vi "日志、报警信息存储 (子VI).vi"() -> ()   [LabVIEW 2016, in "超标留样集成.lvlib" / "ESTD1200.lvlib"]
uses:
  ESTD1200.lvlib
  <vilib>/ptbypt/NI_PtbyPt.lvlib
panel:
  out "采样器状态":u16(ring) items=["空闲", "忙碌"]
  out "状态告警区":T1 {"告警代码" items=["无告警", "通讯异常(采样器与工控机通讯)", "滑台电机异常(过温/过流)", "蠕动泵异常(过温/过流)", "转盘电机异常(过温/过流)", "编码器异常", "转盘原点传感器异常", "滑台原点传感器异常", "冰箱温度异常", "冰箱通讯异常", "门禁锁异常", "串口屏通讯异常", "SD卡异常告警", "Flash异常告警(W25Q32)", "留样失败", "满瓶告警", "复位异常"]; "采样模式" items=["定时采样", "外控采样", "时间等比", "流量等比", "液位等比"]; "当前进程" items=["待机", "电机复位", "采样瓶转到采样区", "采样瓶排空", "采样泵管润洗", "采样瓶再排空", "采样", "采样泵反转排空管路", "取样瓶转到取样区"]}
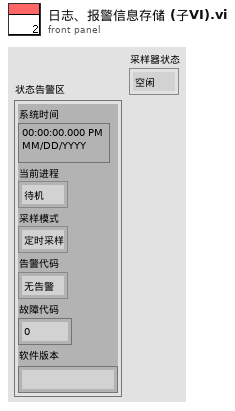
[diagram p1: front panel]
types:
  T1 = cluster{"系统时间":timestamp, "当前进程":u16, "采样模式":u16, "告警代码":u16, "故障代码":u16, "软件版本":string}
  T2 = cluster{"时间标识":timestamp, "设备":string, "日志信息":string, "流程参数":string}
  T3 = cluster{"时间标识":timestamp, "设备":string, "日志信息":string}
  T4 = cluster{"采样器状态":u16, "采样模式":u16, "瓶数":u16, "采样量":u16, "当前瓶号":u16, "当前进程":u16, "采样瓶状态":cluster{"1号瓶":bool, "2号瓶":bool, "3号瓶":bool, "4号瓶":bool, "5号瓶":bool, "6号瓶":bool, "7号瓶":bool, "8号瓶":bool, "9号瓶":bool, "10号瓶":bool, "11号瓶":bool, "12号瓶":bool}, "门锁状态":bool, "冰箱当前温度":sgl, "系统时间":timestamp}
  T5 = cluster{"当前瓶号":u16, "瓶数":u16, "采样量":u16, "采样模式":u16, "整点定时时间":cluster{"1":bool, "2":bool, "3":bool, "4":bool, "5":bool, "6":bool, "7":bool, "8":bool, "9":bool, "10":bool, "11":bool, "12":bool, "13":bool, "14":bool, "15":bool, "16":bool, "17":bool, "19":bool, "19":bool, "20":bool, "21":bool, "22":bool, "23":bool, "24":bool}, "氨氮":sgl, "总磷":sgl, "总氮":sgl, "CODMn":sgl, "CODCr":sgl, "PH":sgl, "溶解氧":sgl, "时间等比采样间隔":u16, "流量等比采样间隔":sgl, "4mA流量":sgl, "20mA流量":sgl, "当前流量":sgl, "液位等比采样间隔":sgl, "4mA液位":sgl, "20mA液位":sgl, "当前液位":sgl}
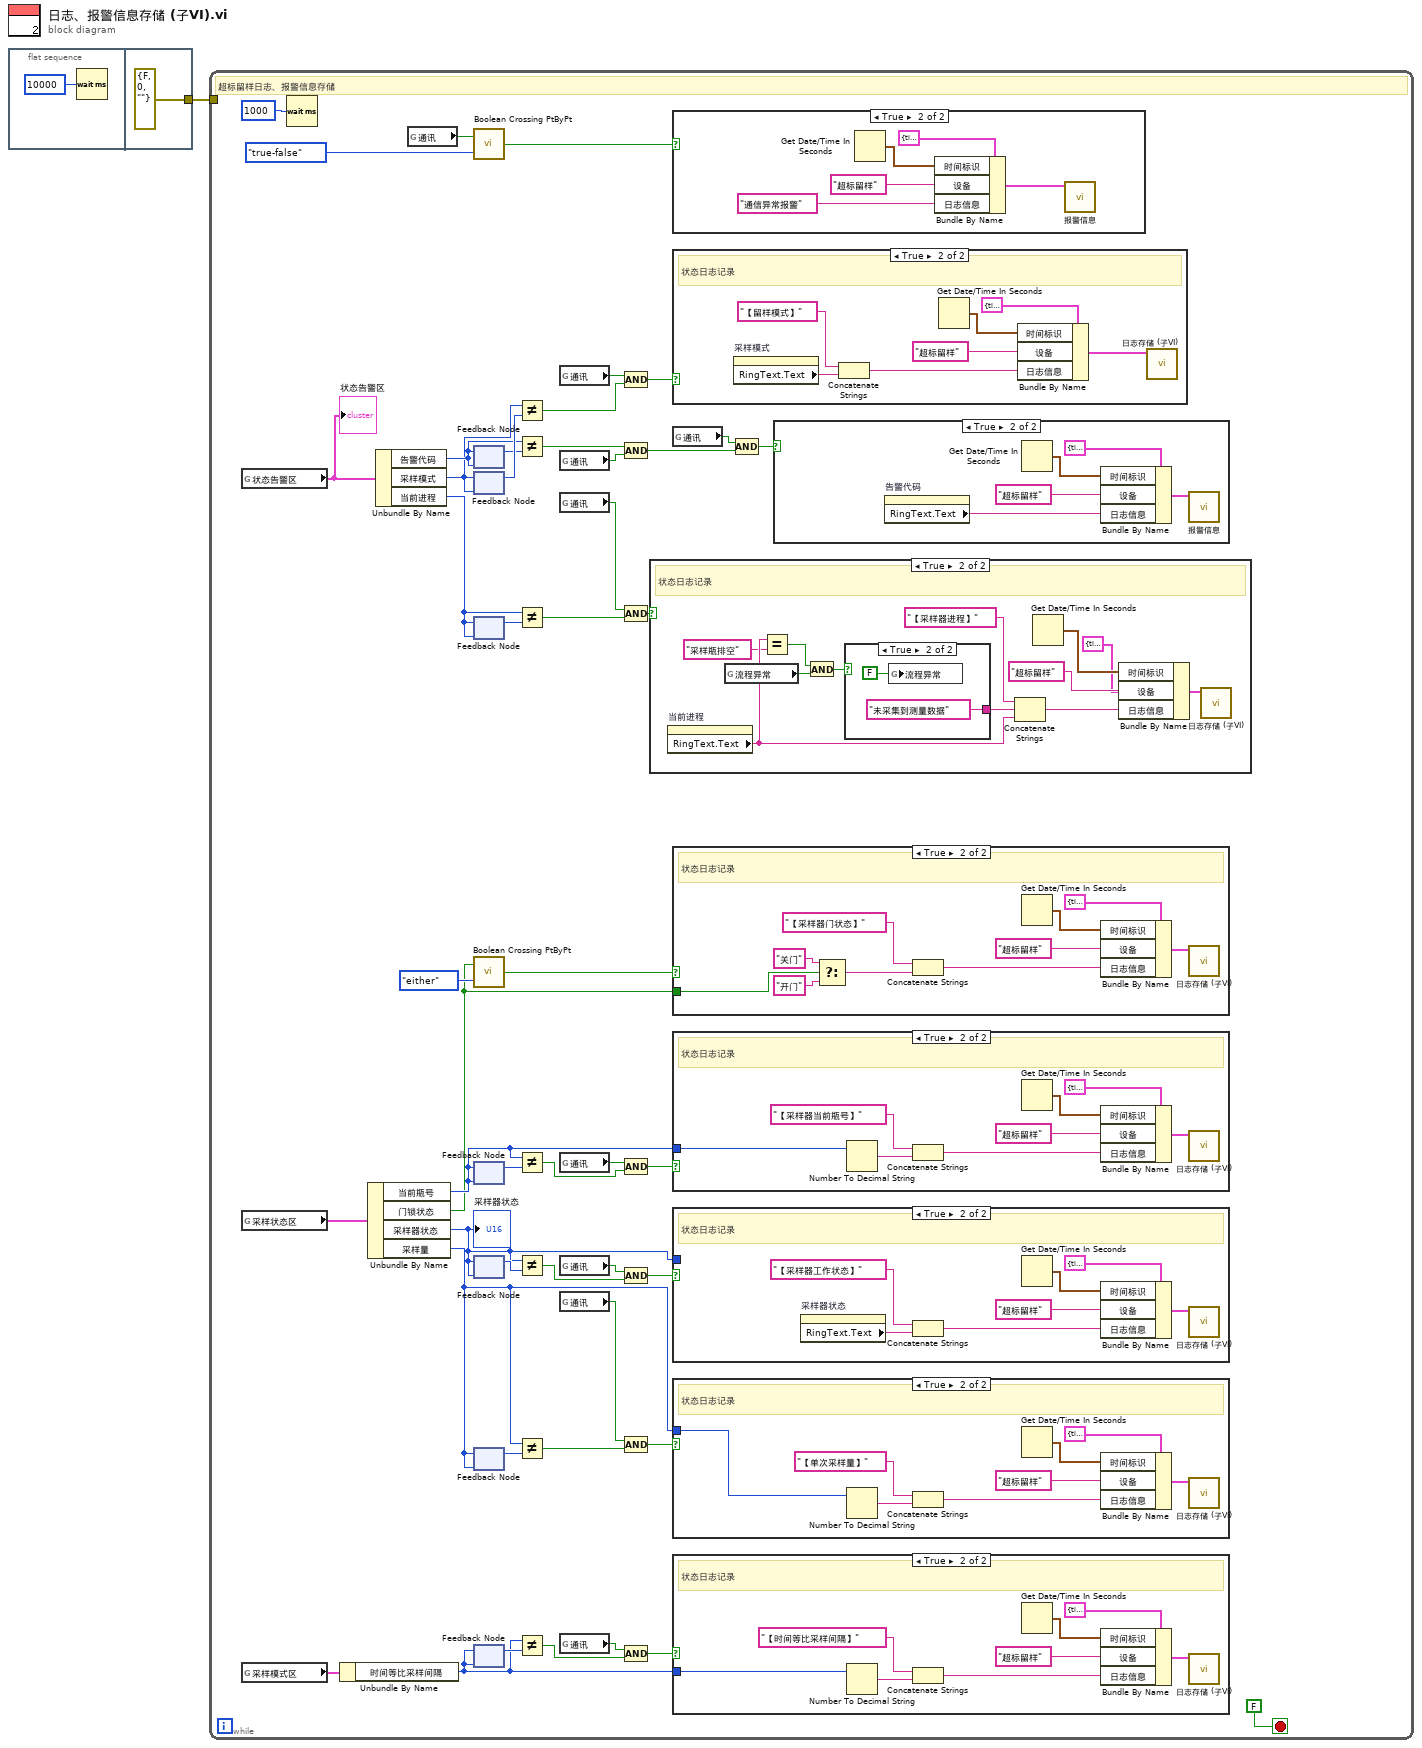
[diagram p0: block diagram]
diagram:
  n1 = flat-sequence {
    tunnel: [errorcluster {"status"=FALSE, "code"=0, "source"=""} ("错误常量")] -> w1
    frame #0 {
      n2 = Wait (ms)(milliseconds to wait=u32 10000 ("等待时间（毫秒）")) -> ()  [unwired: 1 out]
    }
    frame #1 {
    }
  }
  n3 = while {
    tunnel: w1 -> [_]
    stop <- FALSE stop-if-true
    # "超标留样日志、报警信息存储"
    n4 = global read "超标留样全局.vi" "状态告警区"() -> (w16:T1)
    "状态告警区" <- w16
    n5 = global read "超标留样全局.vi" "采样状态区"() -> (w13:T4)
    n6 = global read "超标留样全局.vi" "采样模式区"() -> (w6:T5)
    n7 = Wait (ms)(milliseconds to wait=u32 1000 ("等待时间（毫秒）")) -> ()  [unwired: 1 out]
    n8 = Unbundle By Name(w6) -> ("时间等比采样间隔"=w5:u16)
    n9 = Unbundle By Name(w13) -> ("当前瓶号"=w12:u16, "门锁状态"=w9:bool, "采样器状态"=w8:u16, "采样量"=w7:u16)
    "采样器状态" <- w8
    n10 = Unbundle By Name(w16) -> ("告警代码"=w17:u16, "采样模式"=w15:u16, "当前进程"=w14:u16)
    n11 = global read "超标留样全局.vi" "通讯"() -> (w20:bool)
    n12 = call <vilib>:"Boolean Crossing PtByPt.vi"("direction"=enum16{"either", "false-true", "true-false"}."true-false", "input"=w20) -> ("crossing"=w18:bool)  [unwired: 1 in]
    n13 = feedback #1(w17) -> (w4:u16)
    n14 = feedback-in #1(w17) -> ()
    n15 = feedback #2(w15) -> (w43:u16)
    n16 = feedback-in #2(w15) -> ()
    n17 = feedback #3(w14) -> (w49:u16)
    n18 = feedback-in #3(w14) -> ()
    n19 = call <vilib>:"Boolean Crossing PtByPt.vi"("direction"=enum16{"either", "false-true", "true-false"}."either", "input"=w9) -> ("crossing"=w10:bool)  [unwired: 1 in]
    n20 = feedback #4(w12) -> (w48:u16)
    n21 = feedback-in #4(w12) -> ()
    n22 = feedback #5(w8) -> (w47:u16)
    n23 = feedback-in #5(w8) -> ()
    n24 = feedback #6(w7) -> (w46:u16)
    n25 = feedback-in #6(w7) -> ()
    n26 = feedback #7(w5) -> (w42:u16)
    n27 = feedback-in #7(w5) -> ()
    n28 = Not Equal?(x=w15, y=w43) -> (x != y?=w34:bool)
    n29 = Not Equal?(x=w17, y=w4) -> (x != y?=w39:bool)
    n30 = Not Equal?(x=w14, y=w49) -> (x != y?=w35:bool)
    n31 = Not Equal?(x=w12, y=w48) -> (x != y?=w30:bool)
    n32 = Not Equal?(x=w8, y=w47) -> (x != y?=w28:bool)
    n33 = Not Equal?(x=w7, y=w46) -> (x != y?=w25:bool)
    n34 = Not Equal?(x=w5, y=w42) -> (x != y?=w21:bool)
    n35 = global read "超标留样全局.vi" "通讯"() -> (w38:bool)
    n36 = global read "超标留样全局.vi" "通讯"() -> (w41:bool)
    n37 = global read "超标留样全局.vi" "通讯"() -> (w37:bool)
    n38 = global read "超标留样全局.vi" "通讯"() -> (w32:bool)
    n39 = global read "超标留样全局.vi" "通讯"() -> (w29:bool)
    n40 = global read "超标留样全局.vi" "通讯"() -> (w26:bool)
    n41 = global read "超标留样全局.vi" "通讯"() -> (w23:bool)
    n42 = Compound Arithmetic op=AND ("复合运算")(w38, w34) -> (w33:bool)
    n43 = Compound Arithmetic op=AND ("复合运算")(w39, w41) -> (w40:bool)
    n44 = Compound Arithmetic op=AND ("复合运算")(w37, w35) -> (w36:bool)
    n45 = Compound Arithmetic op=AND ("复合运算")(w32, w30) -> (w31:bool)
    n46 = Compound Arithmetic op=AND ("复合运算")(w29, w28) -> (w27:bool)
    n47 = Compound Arithmetic op=AND ("复合运算")(w26, w25) -> (w24:bool)
    n48 = Compound Arithmetic op=AND ("复合运算")(w23, w21) -> (w22:bool)
    n49 = case shown="True" w36 {
      frame False {
      }
      frame True {
        # "状态日志记录"
        n50 = property on="当前进程" class="Ring (strict)"() -> ("RingText.Text"=w115:string)  [unwired: 2 in, 2 out]
        n51 = global read "串口参数断电保存全局变量.vi" "流程异常"() -> (w112:bool)
        n52 = Equal?(x=w115, y="采样瓶排空") -> (x = y?=w113:bool)
        n53 = And(x=w113, y=w112) -> (x .and. y?=w111:bool)
        n54 = case shown="True" w111 {
          tunnel: [_ "未采集到测量数据" ("t")] -> w110
          frame False {
          }
          frame True {
            n55 = global write "串口参数断电保存全局变量.vi" "流程异常"(FALSE) -> ()
          }
        }
        n56 = Concatenate Strings("【采样器进程】" ("日志信息"), w110, w115) -> (w121:string)
        n57 = Get Date/Time In Seconds() -> (seconds since 1Jan1904=w119:timestamp)
        n58 = Bundle By Name(cluster=T2 {"时间标识"=timestamp(0 s since 1904-01-01), "设备"="", "日志信息"="", "流程参数"=""} ("data in"), "时间标识"=w119, "设备"="超标留样", "日志信息"=w121) -> (w116:T2)
        n59 = call "日志存储 (子VI).vi"("data in"=w116) -> ()  [unwired: 11 in]
      }
    }
    n60 = case shown="True" w18 {
      frame False {
      }
      frame True {
        n61 = Get Date/Time In Seconds() -> (seconds since 1Jan1904=w62:timestamp)
        n62 = Bundle By Name(cluster=T3 {"时间标识"=timestamp(0 s since 1904-01-01), "设备"="", "日志信息"=""} ("data in"), "时间标识"=w62, "设备"="超标留样", "日志信息"="通信异常报警") -> (w66:T3)
        n63 = call "报警信息.vi"("data in"=w66) -> ()  [unwired: 10 in, 1 out]
      }
    }
    n64 = case shown="True" w33 {
      frame False {
      }
      frame True {
        # "状态日志记录"
        n65 = property on="采样模式" class="Ring (strict)"() -> ("RingText.Text"=w75:string)  [unwired: 2 in, 2 out]
        n66 = Concatenate Strings("【留样模式】" ("日志信息"), w75) -> (w81:string)
        n67 = Get Date/Time In Seconds() -> (seconds since 1Jan1904=w78:timestamp)
        n68 = Bundle By Name(cluster=T2 {"时间标识"=timestamp(0 s since 1904-01-01), "设备"="", "日志信息"="", "流程参数"=""} ("data in"), "时间标识"=w78, "设备"="超标留样", "日志信息"=w81) -> (w77:T2)
        n69 = call "日志存储 (子VI).vi"("data in"=w77) -> ()  [unwired: 11 in]
      }
    }
    n70 = global read "超标留样全局.vi" "通讯"() -> (w45:bool)
    n71 = case shown="True" w10 {
      tunnel: w9 -> [_ w55]
      frame False {
      }
      frame True {
        # "状态日志记录"
        n72 = Select(t="关门", s=w55, f="开门") -> (s? t:f=w52:string)
        n73 = Concatenate Strings("【采样器门状态】" ("日志信息"), w52) -> (w61:string)
        n74 = Get Date/Time In Seconds() -> (seconds since 1Jan1904=w58:timestamp)
        n75 = Bundle By Name(cluster=T2 {"时间标识"=timestamp(0 s since 1904-01-01), "设备"="", "日志信息"="", "流程参数"=""} ("data in"), "时间标识"=w58, "设备"="超标留样", "日志信息"=w61) -> (w57:T2)
        n76 = call "日志存储 (子VI).vi"("data in"=w57) -> ()  [unwired: 11 in]
      }
    }
    n77 = case shown="True" w31 {
      tunnel: w12 -> [_ w103]
      frame False {
      }
      frame True {
        # "状态日志记录"
        n78 = Number To Decimal String(number=w103) -> (decimal integer string=w102:string)  [unwired: 1 in]
        n79 = Concatenate Strings("【采样器当前瓶号】" ("日志信息"), w102) -> (w109:string)
        n80 = Get Date/Time In Seconds() -> (seconds since 1Jan1904=w106:timestamp)
        n81 = Bundle By Name(cluster=T2 {"时间标识"=timestamp(0 s since 1904-01-01), "设备"="", "日志信息"="", "流程参数"=""} ("data in"), "时间标识"=w106, "设备"="超标留样", "日志信息"=w109) -> (w105:T2)
        n82 = call "日志存储 (子VI).vi"("data in"=w105) -> ()  [unwired: 11 in]
      }
    }
    n83 = case shown="True" w27 {
      tunnel: w8 -> [_ _]
      frame False {
      }
      frame True {
        # "状态日志记录"
        n84 = property on="采样器状态" class="Ring (strict)"() -> ("RingText.Text"=w95:string)  [unwired: 2 in, 2 out]
        n85 = Concatenate Strings("【采样器工作状态】" ("日志信息"), w95) -> (w101:string)
        n86 = Get Date/Time In Seconds() -> (seconds since 1Jan1904=w98:timestamp)
        n87 = Bundle By Name(cluster=T2 {"时间标识"=timestamp(0 s since 1904-01-01), "设备"="", "日志信息"="", "流程参数"=""} ("data in"), "时间标识"=w98, "设备"="超标留样", "日志信息"=w101) -> (w97:T2)
        n88 = call "日志存储 (子VI).vi"("data in"=w97) -> ()  [unwired: 11 in]
      }
    }
    n89 = case shown="True" w24 {
      tunnel: w7 -> [_ w88]
      frame False {
      }
      frame True {
        # "状态日志记录"
        n90 = Number To Decimal String(number=w88) -> (decimal integer string=w87:string)  [unwired: 1 in]
        n91 = Concatenate Strings("【单次采样量】" ("日志信息"), w87) -> (w94:string)
        n92 = Get Date/Time In Seconds() -> (seconds since 1Jan1904=w91:timestamp)
        n93 = Bundle By Name(cluster=T2 {"时间标识"=timestamp(0 s since 1904-01-01), "设备"="", "日志信息"="", "流程参数"=""} ("data in"), "时间标识"=w91, "设备"="超标留样", "日志信息"=w94) -> (w90:T2)
        n94 = call "日志存储 (子VI).vi"("data in"=w90) -> ()  [unwired: 11 in]
      }
    }
    n95 = case shown="True" w22 {
      tunnel: w5 -> [_ w68]
      frame False {
      }
      frame True {
        # "状态日志记录"
        n96 = Number To Decimal String(number=w68) -> (decimal integer string=w67:string)  [unwired: 1 in]
        n97 = Concatenate Strings("【时间等比采样间隔】" ("日志信息"), w67) -> (w74:string)
        n98 = Get Date/Time In Seconds() -> (seconds since 1Jan1904=w71:timestamp)
        n99 = Bundle By Name(cluster=T2 {"时间标识"=timestamp(0 s since 1904-01-01), "设备"="", "日志信息"="", "流程参数"=""} ("data in"), "时间标识"=w71, "设备"="超标留样", "日志信息"=w74) -> (w70:T2)
        n100 = call "日志存储 (子VI).vi"("data in"=w70) -> ()  [unwired: 11 in]
      }
    }
    n101 = Compound Arithmetic op=AND ("复合运算")(w45, w40) -> (w44:bool)
    n102 = case shown="True" w44 {
      frame False {
      }
      frame True {
        n103 = property on="告警代码" class="Ring (strict)"() -> ("RingText.Text"=w82:string)  [unwired: 2 in, 2 out]
        n104 = Get Date/Time In Seconds() -> (seconds since 1Jan1904=w86:timestamp)
        n105 = Bundle By Name(cluster=T3 {"时间标识"=timestamp(0 s since 1904-01-01), "设备"="", "日志信息"=""} ("data in"), "时间标识"=w86, "设备"="超标留样", "日志信息"=w82) -> (w83:T3)
        n106 = call "报警信息.vi"("data in"=w83) -> ()  [unwired: 10 in, 1 out]
      }
    }
  }
